vi "TSM_read_hex_data.vi"(8 "error in (no error)":errorcluster, 11 "read buffer in":string) -> (0 "error out":errorcluster, 1 "Terminator":string, 2 "SensorData":T1, 3 "Position":T2)   [LabVIEW 2020]
uses:
  Position_TypDef.ctl
  SensorData_TypDef.ctl
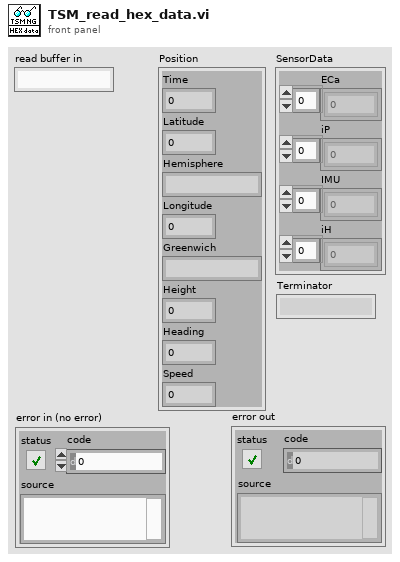
[diagram p1: front panel]
types:
  T1 = typedef "SensorData_TypDef.ctl" = cluster{"ECa":dbl[], "iP":dbl[], "IMU":dbl[], "iH":dbl[]}
  T2 = typedef "Position_TypDef.ctl" = cluster{"Time":u32, "Latitude":u32, "Hemisphere":string, "Longitude":u32, "Greenwich":string, "Height":u32, "Heading":u32, "Speed":u32}
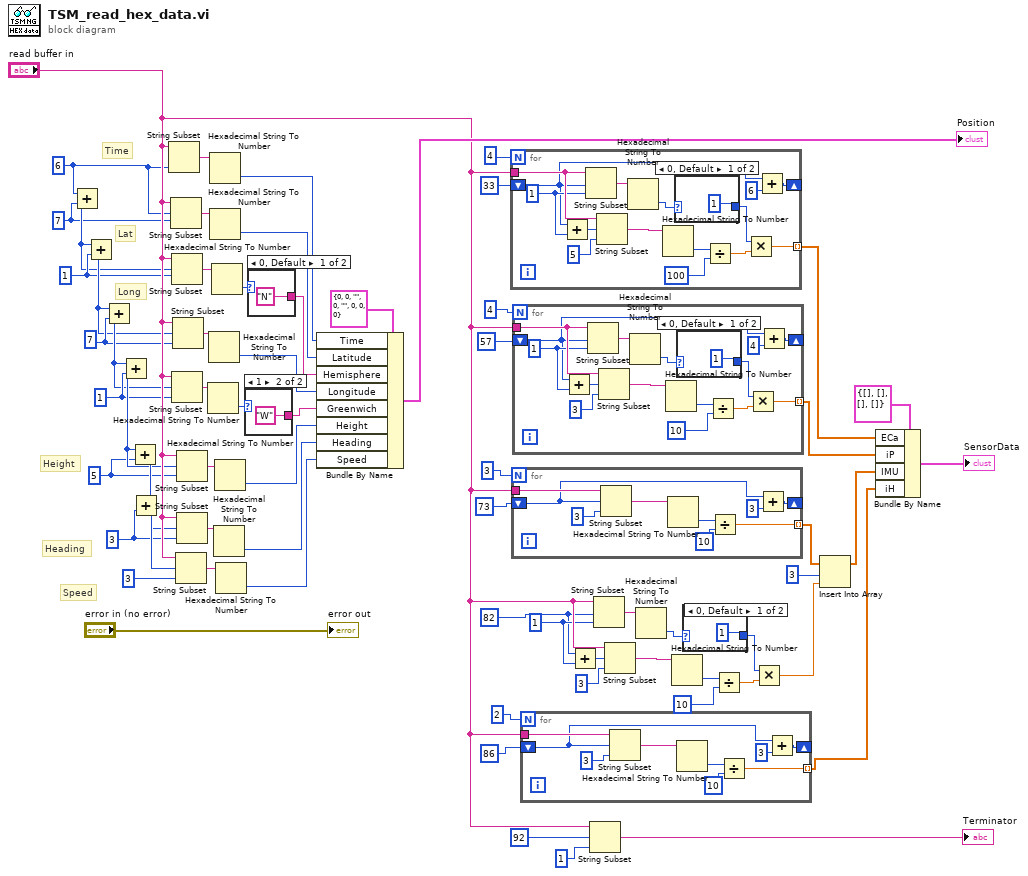
[diagram p0: block diagram]
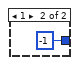
[diagram p2: hidden frame]
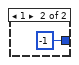
[diagram p3: hidden frame]
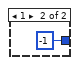
[diagram p4: hidden frame]
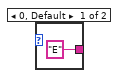
[diagram p5: hidden frame]
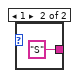
[diagram p6: hidden frame]
diagram:
  w34 = 1
  w32 = 82
  w22 = 3
  w18 = 5
  w16 = 1
  w12 = 7
  w9 = 1
  w4 = 7
  w5 = 6
  # "Time"
  # "Lat"
  # "Long"
  # "Speed"
  # "Heading"
  # "Height"
  n1 = Add(x=w5, y=w4) -> (x+y=w8:i32)
  n2 = Add(x=w8, y=w9) -> (x+y=w11:i32)
  n3 = Add(x=w11, y=w12) -> (x+y=w15:i32)
  n4 = Add(x=w15, y=w16) -> (x+y=w19:i32)
  n5 = Add(x=w19, y=w18) -> (x+y=w21:i32)
  n6 = Add(x=w21, y=w22) -> (x+y=w24:i32)
  n7 = String Subset(string="read buffer in", length (rest)=w5) -> (substring=w2:string)  [unwired: 1 in]
  n8 = String Subset(string="read buffer in", offset (0)=w5, length (rest)=w4) -> (substring=w3:string)
  n9 = String Subset(string="read buffer in", offset (0)=w8, length (rest)=w9) -> (substring=w6:string)
  n10 = String Subset(string="read buffer in", offset (0)=w15, length (rest)=w16) -> (substring=w13:string)
  n11 = String Subset(string="read buffer in", offset (0)=w11, length (rest)=w12) -> (substring=w10:string)
  n12 = String Subset(string="read buffer in", offset (0)=w24, length (rest)=3) -> (substring=w23:string)
  n13 = String Subset(string="read buffer in", offset (0)=w19, length (rest)=w18) -> (substring=w17:string)
  n14 = String Subset(string="read buffer in", offset (0)=w21, length (rest)=w22) -> (substring=w20:string)
  n15 = Hexadecimal String To Number(string=w13) -> (number=w14:u32)  [unwired: 2 in, 1 out]
  n16 = Hexadecimal String To Number(string=w10) -> (number=w57:u32)  [unwired: 2 in, 1 out]
  n17 = Hexadecimal String To Number(string=w2) -> (number=w60:u32)  [unwired: 2 in, 1 out]
  n18 = Hexadecimal String To Number(string=w3) -> (number=w59:u32)  [unwired: 2 in, 1 out]
  n19 = Hexadecimal String To Number(string=w6) -> (number=w7:u32)  [unwired: 2 in, 1 out]
  n20 = Hexadecimal String To Number(string=w20) -> (number=w54:u32)  [unwired: 2 in, 1 out]
  n21 = Hexadecimal String To Number(string=w17) -> (number=w55:u32)  [unwired: 2 in, 1 out]
  n22 = Hexadecimal String To Number(string=w23) -> (number=w53:u32)  [unwired: 2 in, 1 out]
  n23 = case shown="1" w14 {
    tunnel: ["E" "W"] -> w56
    frame 0, Default {
    }
    frame 1 {
    }
  }
  n24 = case shown="0, Default" w7 {
    tunnel: ["N" "S"] -> w58
    frame 0, Default {
    }
    frame 1 {
    }
  }
  n25 = Bundle By Name(cluster=T2 {"Time"=0, "Latitude"=0, "Hemisphere"="", "Longitude"=0, "Greenwich"="", "Height"=0, "Heading"=0, "Speed"=0} ("Position"), "Time"=w60, "Latitude"=w59, "Hemisphere"=w58, "Longitude"=w57, "Greenwich"=w56, "Height"=w55, "Heading"=w54, "Speed"=w53) -> (→"Position":T2)
  n26 = for {
    N: 4 -> [_]
    tunnel: "read buffer in" -> [w86]
    shift-right: [w75] -> _
    shift-left: 33 -> [w74]
    tunnel: [w72] -> w62 mode=indexing
    w84 = 1
    n27 = Add(x=w74, y=w84) -> (x+y=w85:i32)
    n28 = String Subset(string=w86, offset (0)=w74, length (rest)=w84) -> (substring=w82:string)
    n29 = String Subset(string=w86, offset (0)=w85, length (rest)=5) -> (substring=w81:string)
    n30 = Hexadecimal String To Number(string=w82) -> (number=w78:u32)  [unwired: 2 in, 1 out]
    n31 = Hexadecimal String To Number(string=w81) -> (number=w80:u32)  [unwired: 2 in, 1 out]
    n32 = case shown="0, Default" w78 {
      tunnel: [1 -1] -> w77
      frame 0, Default {
      }
      frame 1 {
      }
    }
    n33 = Divide(x=w80, y=100) -> (x/y=w76:dbl)
    n34 = Multiply(x=w77, y=w76) -> (x*y=w72:dbl)
    n35 = Add(x=w74, y=6) -> (x+y=w75:i32)
  }
  n36 = for {
    N: 3 -> [_]
    tunnel: "read buffer in" -> [w97]
    shift-right: [w92] -> _
    shift-left: 73 -> [w89]
    tunnel: [w90] -> w43 mode=indexing
    n37 = String Subset(string=w97, offset (0)=w89, length (rest)=3) -> (substring=w95:string)
    n38 = Hexadecimal String To Number(string=w95) -> (number=w94:u32)  [unwired: 2 in, 1 out]
    n39 = Divide(x=w94, y=10) -> (x/y=w90:dbl)
    n40 = Add(x=w89, y=3) -> (x+y=w92:i32)
  }
  n41 = for {
    N: 4 -> [_]
    tunnel: "read buffer in" -> [w112]
    shift-right: [w101] -> _
    shift-left: 57 -> [w100]
    tunnel: [w98] -> w63 mode=indexing
    w110 = 1
    n42 = Add(x=w100, y=w110) -> (x+y=w111:i32)
    n43 = String Subset(string=w112, offset (0)=w100, length (rest)=w110) -> (substring=w108:string)
    n44 = String Subset(string=w112, offset (0)=w111, length (rest)=3) -> (substring=w107:string)
    n45 = Hexadecimal String To Number(string=w108) -> (number=w104:u32)  [unwired: 2 in, 1 out]
    n46 = Hexadecimal String To Number(string=w107) -> (number=w106:u32)  [unwired: 2 in, 1 out]
    n47 = case shown="0, Default" w104 {
      tunnel: [1 -1] -> w103
      frame 0, Default {
      }
      frame 1 {
      }
    }
    n48 = Divide(x=w106, y=10) -> (x/y=w102:dbl)
    n49 = Multiply(x=w103, y=w102) -> (x*y=w98:dbl)
    n50 = Add(x=w100, y=4) -> (x+y=w101:i32)
  }
  n51 = for {
    N: 2 -> [_]
    tunnel: "read buffer in" -> [w123]
    shift-right: [w118] -> _
    shift-left: 86 -> [w115]
    tunnel: [w116] -> w65 mode=indexing
    n52 = String Subset(string=w123, offset (0)=w115, length (rest)=3) -> (substring=w121:string)
    n53 = Hexadecimal String To Number(string=w121) -> (number=w120:u32)  [unwired: 2 in, 1 out]
    n54 = Divide(x=w120, y=10) -> (x/y=w116:dbl)
    n55 = Add(x=w115, y=3) -> (x+y=w118:i32)
  }
  n56 = Add(x=w32, y=w34) -> (x+y=w33:i32)
  n57 = String Subset(string="read buffer in", offset (0)=92, length (rest)=1) -> (substring=→"Terminator":string)
  n58 = String Subset(string="read buffer in", offset (0)=w32, length (rest)=w34) -> (substring=w36:string)
  n59 = String Subset(string="read buffer in", offset (0)=w33, length (rest)=3) -> (substring=w37:string)
  n60 = Hexadecimal String To Number(string=w36) -> (number=w40:u32)  [unwired: 2 in, 1 out]
  n61 = Hexadecimal String To Number(string=w37) -> (number=w38:u32)  [unwired: 2 in, 1 out]
  n62 = case shown="0, Default" w40 {
    tunnel: [1 -1] -> w41
    frame 0, Default {
    }
    frame 1 {
    }
  }
  n63 = Divide(x=w38, y=10) -> (x/y=w42:dbl)
  n64 = Multiply(x=w41, y=w42) -> (x*y=w45:dbl)
  n65 = Insert Into Array(array=w43, index=3, new element=w45) -> (w64:dbl[])
  n66 = Bundle By Name(cluster=T1 {"ECa"=[], "iP"=[], "IMU"=[], "iH"=[]} ("SensorData"), "ECa"=w62, "iP"=w63, "IMU"=w64, "iH"=w65) -> (→"SensorData":T1)
  "error out" <- "error in (no error)"
